vi "AnalogOutput-Command string parser.vi"(3 "error in":errorcluster, 5 "Command string":string) -> (0 "error out":errorcluster, 2 "Waveform":waveform(dbl))   [LabVIEW 2015]
doc: "Parses an AnalogOutput command string.\n\nCurrently only supports sine waves.\nThese should look something like:\nsine;2000Hz;1.2V;250ms;sample100000Hz;"
uses:
  Typedefs/AnalogOutput_SineSequence.ctl
  Typedefs/AnalogOutput_SquareSequence.ctl
  <vilib>/Waveform/WDTOps.llb/WDT Append Waveforms DBL.vi
  <vilib>/measure/NI_MABase.lvlib
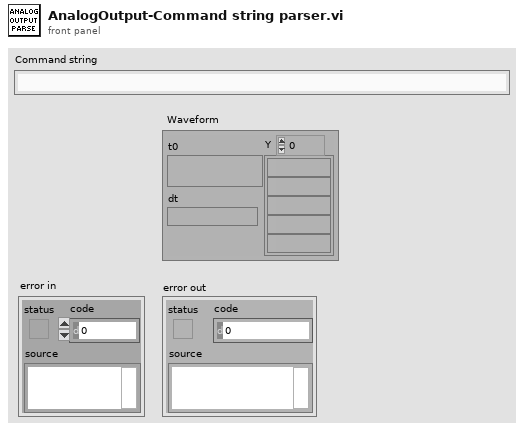
[diagram p1: front panel]
types:
  T1 = enum16{"Sine Wave", "Triangle Wave", "Square Wave", "Sawtooth Wave"}
  T2 = typedef "AnalogOutput_SineSequence.ctl" = cluster{"Frequency (Hz)":dbl, "Duration (ms)":dbl, "Amplitude (V)":dbl, "Sample clock (Hz)":dbl}[]
  T3 = typedef "AnalogOutput_SquareSequence.ctl" = cluster{"Frequency (Hz)":dbl, "Duty Cycle":dbl, "Duration (ms)":dbl, "Sample clock (Hz)":dbl, "Amplitude (V)":dbl}[]
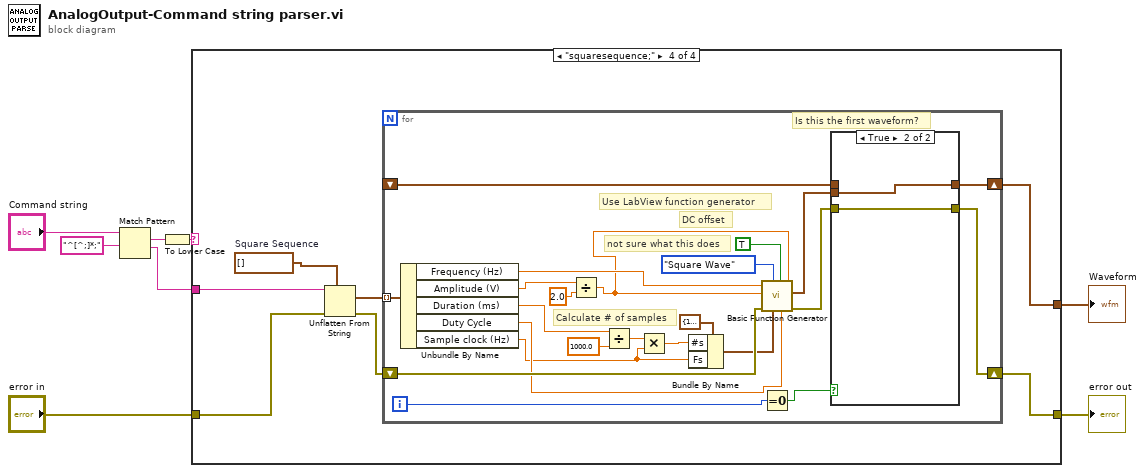
[diagram p0: block diagram]
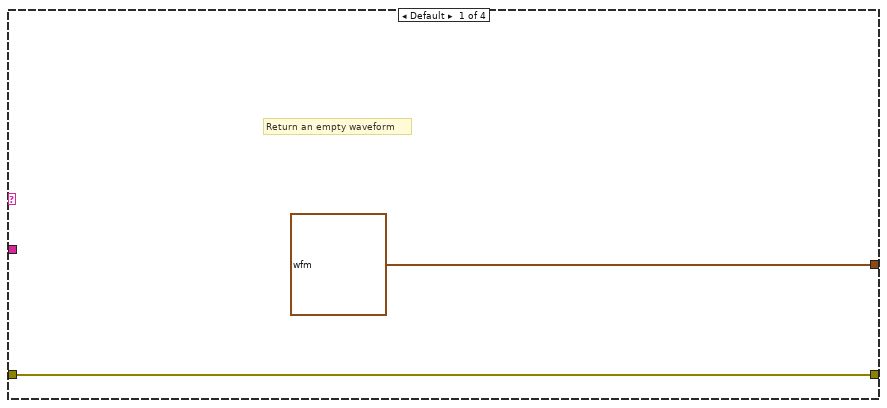
[diagram p2: hidden frame]
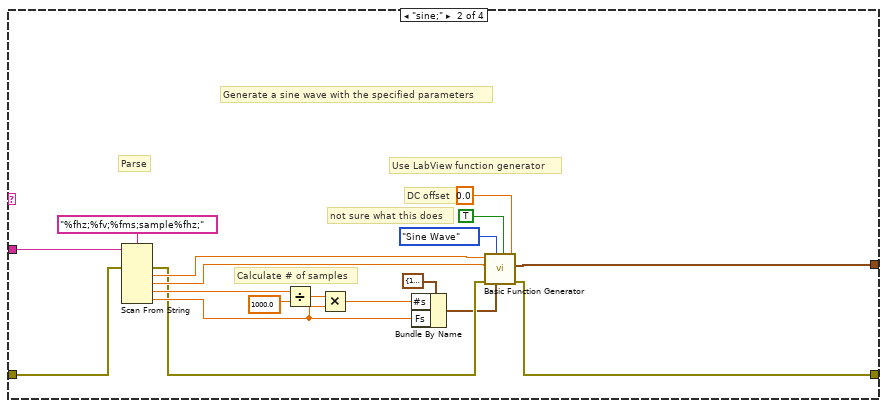
[diagram p3: hidden frame]
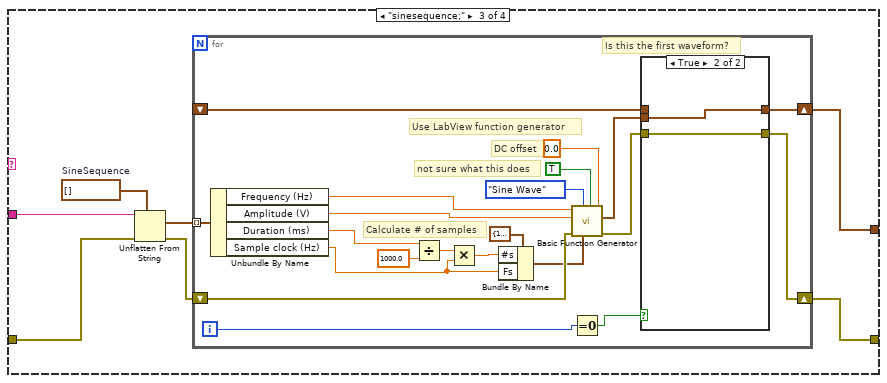
[diagram p4: hidden frame]
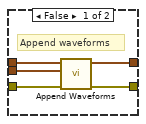
[diagram p5: hidden frame]
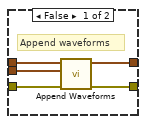
[diagram p6: hidden frame]
diagram:
  n1 = Match Pattern(string="Command string", regular expression="^[^;]*;") -> (match substring=w5:string, after substring=w1:string)  [unwired: 1 in, 2 out]
  n2 = To Lower Case(string=w5) -> (all lower case string=w4:string)
  n3 = case shown="\"squaresequence;\"" w4 {
    tunnel: w1 -> [_ w27 w35 w68]
    tunnel: "error in" -> [w9 w26 w33 w67]
    tunnel: [w9 w15 w29 w65] -> w7
    tunnel: [waveform(dbl) {"t0"=timestamp(0 s since 1904-01-01), "dt"=0.0, "Y"=[]} ("Waveform") w14 w30 w66] -> w6
    frame Default {
      # "Return an empty waveform"
    }
    frame "sine;" {
      # "Use LabView function generator"
      # "Calculate # of samples"
      # "Parse"
      # "Generate a sine wave with the specified parameters"
      # "DC offset"
      # "not sure what this does"
      n4 = Scan From String(format string="%fhz;%fv;%fms;sample%fhz;", input string=w27, error in=w26) -> (error out=w17:errorcluster, output 1=w19:dbl, output 2=w18:dbl, output 3=w24:dbl, output 4=w25:dbl)  [unwired: 5 in, 2 out]
      n5 = Divide(x=w24, y=1000.0) -> (x/y=w21:dbl)
      n6 = Multiply(x=w21, y=w25) -> (x*y=w20:dbl)
      n7 = Bundle By Name(cluster=cluster{"Fs":dbl, "#s":dbl} {"Fs"=1000.0, "#s"=1000.0} ("sampling info"), "#s"=w20, "Fs"=w25) -> (w16:cluster{"Fs":dbl, "#s":dbl})
      n8 = call <vilib>:"Basic Function Generator.vi"("offset"=0.0, "reset signal"=TRUE, "sampling info"=w16, "signal type"=T1."Sine Wave", "error in (no error)"=w17, "amplitude"=w18, "frequency"=w19) -> ("error out"=w15:errorcluster, "signal out"=w14:waveform(dbl))  [unwired: 2 in, 1 out]
    }
    frame "sinesequence;" {
      w34 = T2 []  # SineSequence
      n9 = Unflatten From String(type=w34, binary string=w35, error in (no error)=w33) -> (value=w32:T2, error out=w31:errorcluster)  [unwired: 2 in, 1 out]
      n10 = for {
        tunnel: w32 -> [w55] mode=indexing
        shift-right: [w47] -> w29
        shift-left: w31 -> [w40]
        shift-right: [w48] -> w30
        shift-left: _ -> [w49]
        i -> [w46]
        # "Is this the first waveform?"
        # "Calculate # of samples"
        # "Use LabView function generator"
        # "DC offset"
        # "not sure what this does"
        n11 = Unbundle By Name(w55) -> ("Frequency (Hz)"=w42:dbl, "Amplitude (V)"=w41:dbl, "Duration (ms)"=w52:dbl, "Sample clock (Hz)"=w51:dbl)
        n12 = Divide(x=w52, y=1000.0) -> (x/y=w53:dbl)
        n13 = Multiply(x=w53, y=w51) -> (x*y=w50:dbl)
        n14 = Bundle By Name(cluster=cluster{"Fs":dbl, "#s":dbl} {"Fs"=1000.0, "#s"=1000.0} ("sampling info"), "#s"=w50, "Fs"=w51) -> (w39:cluster{"Fs":dbl, "#s":dbl})
        n15 = call <vilib>:"Basic Function Generator.vi"("offset"=0.0, "reset signal"=TRUE, "sampling info"=w39, "signal type"=T1."Sine Wave", "error in (no error)"=w40, "amplitude"=w41, "frequency"=w42) -> ("error out"=w44:errorcluster, "signal out"=w43:waveform(dbl))  [unwired: 2 in, 1 out]
        n16 = Equal To 0?(x=w46) -> (x = 0?=w45:bool)
        n17 = case shown="True" w45 {
          tunnel: w49 -> [w61 _]
          tunnel: w43 -> [w60 w63]
          tunnel: [w59 w63] -> w48
          tunnel: w44 -> [w58 w62]
          tunnel: [w57 w62] -> w47
          frame False {
            # "Append waveforms"
            n18 = call-poly <vilib>:"Append Waveforms.vi"("error in (no error)"=w58, "waveform B"=w60, "waveform A"=w61) -> ("error out"=w57:errorcluster, "waveform out"=w59:waveform(dbl))  [unwired: 7 in]
          }
          frame True {
          }
        }
      }
    }
    frame "squaresequence;" {
      w64 = T3 []  # Square Sequence
      n19 = Unflatten From String(type=w64, binary string=w68, error in (no error)=w67) -> (value=w70:T3, error out=w69:errorcluster)  [unwired: 2 in, 1 out]
      n20 = for {
        tunnel: w70 -> [w92] mode=indexing
        shift-right: [w85] -> w65
        shift-left: w69 -> [w79]
        shift-right: [w86] -> w66
        shift-left: _ -> [w87]
        i -> [w84]
        # "Is this the first waveform?"
        # "Calculate # of samples"
        # "Use LabView function generator"
        # "DC offset"
        # "not sure what this does"
        n21 = Unbundle By Name(w92) -> ("Frequency (Hz)"=w80:dbl, "Amplitude (V)"=w73:dbl, "Duration (ms)"=w89:dbl, "Duty Cycle"=w75:dbl, "Sample clock (Hz)"=w74:dbl)
        n22 = Divide(x=w73, y=2.0 ("offset")) -> (x/y=w72:dbl)
        n23 = Divide(x=w89, y=1000.0) -> (x/y=w90:dbl)
        n24 = Multiply(x=w90, y=w74) -> (x*y=w88:dbl)
        n25 = Bundle By Name(cluster=cluster{"Fs":dbl, "#s":dbl} {"Fs"=1000.0, "#s"=1000.0} ("sampling info"), "#s"=w88, "Fs"=w74) -> (w78:cluster{"Fs":dbl, "#s":dbl})
        n26 = call <vilib>:"Basic Function Generator.vi"("offset"=w72, "square wave duty cycle (%)"=w75, "reset signal"=TRUE, "sampling info"=w78, "signal type"=T1."Square Wave", "error in (no error)"=w79, "amplitude"=w72, "frequency"=w80) -> ("error out"=w82:errorcluster, "signal out"=w81:waveform(dbl))  [unwired: 1 in, 1 out]
        n27 = Equal To 0?(x=w84) -> (x = 0?=w83:bool)
        n28 = case shown="True" w83 {
          tunnel: w87 -> [w98 _]
          tunnel: w81 -> [w97 w100]
          tunnel: [w96 w100] -> w86
          tunnel: w82 -> [w95 w99]
          tunnel: [w94 w99] -> w85
          frame False {
            # "Append waveforms"
            n29 = call-poly <vilib>:"Append Waveforms.vi"("error in (no error)"=w95, "waveform B"=w97, "waveform A"=w98) -> ("error out"=w94:errorcluster, "waveform out"=w96:waveform(dbl))  [unwired: 7 in]
          }
          frame True {
          }
        }
      }
    }
  }
  "Waveform" <- w6
  "error out" <- w7
